vi "Application_CalcWaitWithEWMA.vi"(5 "DesiredLoopTime[ms]":dbl=30.0 format="%#_13g", 7 "Weight[0-1]":dbl=0.001 min=0.0001 max=0.9999 step=0.0001 format="%#_13g", 11 "LastLoopTime[ms]":dbl format="%#_13g") -> (3 "WaitTime[ms]":u32)   [LabVIEW 2016]
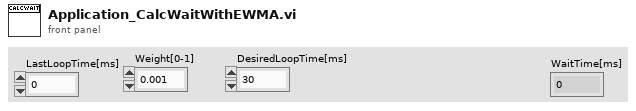
[diagram p1: front panel]
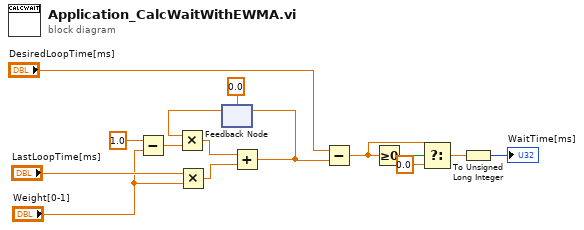
[diagram p0: block diagram]
diagram:
  n1 = Subtract(x=1.0, y="Weight[0-1]") -> (x-y=w12:dbl)
  n2 = Multiply(x="LastLoopTime[ms]", y="Weight[0-1]") -> (x*y=w10:dbl)
  n3 = feedback #1(0.0 ("InitialValue")) -> (w9:dbl)
  n4 = Multiply(x=w9, y=w12) -> (x*y=w11:dbl)
  n5 = Add(x=w11, y=w10) -> (x+y=w2:dbl)
  n6 = feedback-in #1(w2) -> ()
  n7 = Subtract(x="DesiredLoopTime[ms]", y=w2) -> (x-y=w5:dbl)
  n8 = Greater Or Equal To 0?(x=w5) -> (x >= 0?=w6:bool)
  n9 = Select(t=w5, s=w6, f=0.0) -> (s? t:f=w3:dbl)
  n10 = To Unsigned Long Integer(number=w3) -> (unsigned 32bit integer=→"WaitTime[ms]":u32)
